vi "setTypeAndPath.vi"(0 "reference in":refnum<class "File Controller.lvclass">, 2 "file_type":T1, 3 "file_path":path, 5 "error in (no error)":errorcluster) -> (14 "reference out":refnum<class "File Controller.lvclass">, 19 "error out":errorcluster)   [LabVIEW 2015, in "File Controller.lvclass"]
uses:
  File Controller.lvclass
  APP/excelFile_class/fileType.ctl
  APP/excelFile_class/excelFile.lvclass
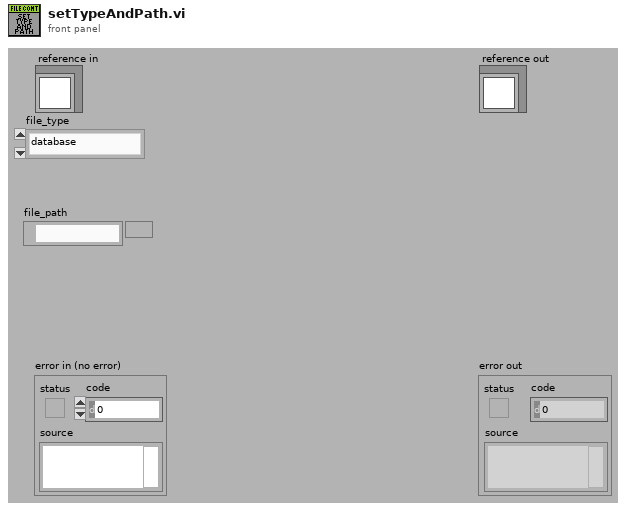
[diagram p1: front panel]
types:
  T1 = typedef "excelFile.lvclass/fileType.ctl" = enum16{"database", "CosmedTest PFTSUITE", "CosmedTest OMNIA"}
  T2 = typedef "File Controller.lvclass/ObjectAttributesRef.ctl" = refnum<data-value>
  T3 = typedef "File Controller.lvclass/ObjectAttributes.ctl" = cluster{"MyAttribute":dbl, "file_path":path, "file_type":T1, "data":string[][][], "excel_file_ref":refnum<class "excelFile.lvclass">, "sheetName":string[], "subject_refs":refnum<class "subject.lvclass">[], "temp_data":string[][][]}
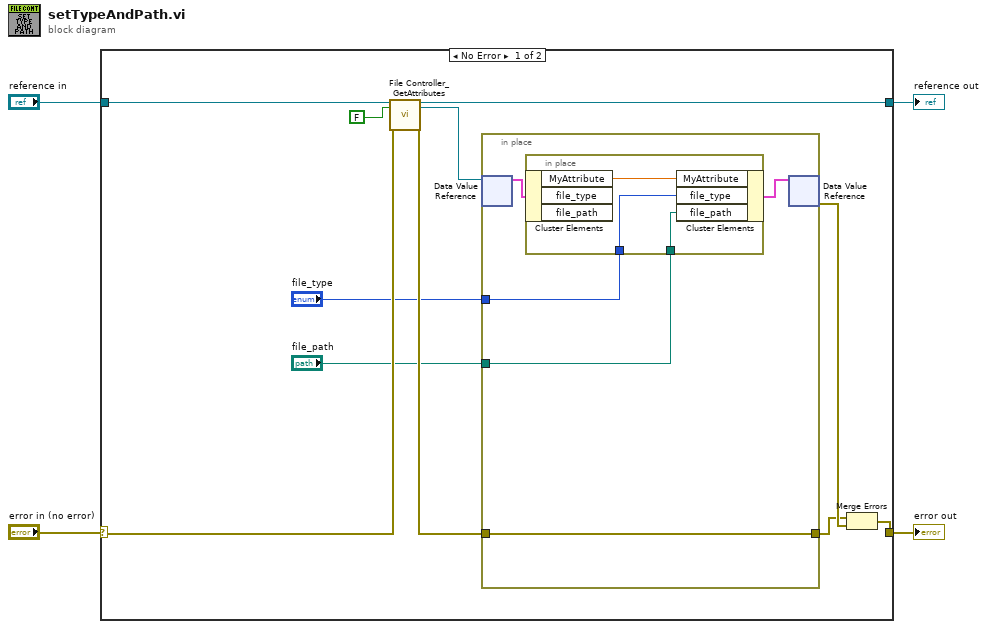
[diagram p0: block diagram]
diagram:
  n1 = case shown="No Error" "error in (no error)" {
    selector: "error in (no error)" -> [w10 w25]
    tunnel: [w15 w25] -> w3
    tunnel: [w8 w24] -> w1
    tunnel: "reference in" -> [w12 w24]
    frame No Error {
      n2 = call "File Controller_GetAttributes.vi"("reference in"=w12, "return data? (T)"=FALSE, "error in (no error)"=w10) -> ("reference out"=w8:refnum<class "File Controller.lvclass">, "attributes ref"=w7:T2, "error out"=w9:errorcluster)  [unwired: 13 in, 1 out]
      n3 = in-place {
        in-place-border: w9 -> [w18]
        in-place-border: [w18] -> w13
        in-place-border: "file_type" -> [w17]
        in-place-border: "file_path" -> [w16]
        n4 = in-place-dvr #1(w7) -> (w19:T3)  [unwired: 1 out]
        n5 = in-place {
          in-place-border: w17 -> [w22]
          in-place-border: w16 -> [w21]
          n6 = in-place-cluster #2(w19) -> ("MyAttribute"=w23:dbl)  [unwired: 2 out]
          n7 = in-place-cluster #2("MyAttribute"=w23, "file_type"=w22, "file_path"=w21) -> (w20:T3)
        }
        n8 = in-place-dvr #1(w20) -> (w14:errorcluster)  [unwired: 1 out]
      }
      n9 = Merge Errors(w13, w14) -> (w15:errorcluster)
    }
    frame Error {
    }
  }
  "error out" <- w3
  "reference out" <- w1
